vi "Peak Detector Comparison.vi"() -> ()   [LabVIEW 2020]
doc: "This VI compares the use of the Peak Detector.vi and the Peak Detector PtByPt.vi and how to use both VIs for the same problem. It also demonstrates how to use Data Queue PtByPt.vi to allow the function Peak Detector to work as a \"sliding window\" to find the location, amplitude, and second derivative of peaks or valleys in the set of generated input data."
uses:
  <vilib>/Analysis/1siggen.llb/Ramp Pattern by Samples.vi
  <vilib>/ptbypt/NI_PtbyPt.lvlib
  <vilib>/Analysis/NI_AALBase.lvlib
panel:
  in  "Motor Enable":bool
  out "First Peak":bool
  out "Motor":bool
  out "peak 2":bool
  in  "Noise Amplitude 2":dbl=1.0
  in  "Width 2":i32(slide)=10 min=3 scale=3.0..20.0
  in  "Sine Wave Amplitude 2":dbl=10.0
  out "peak":bool
  in  "Noise Amplitude":dbl=1.0
  in  "Stop":bool
  in  "Sine Wave Amplitude":dbl=10.0
  out "Signal Input and Peaks/Valleys from Peak Detector":cluster{"Locations":dbl[], "Amplitudes":dbl[]}[](graph)
  in  "Width":i32(slide)=10 min=3 scale=3.0..20.0
  in  "threshold":dbl(slide) scale=-15.0..15.0
  # "PtByPt Results"
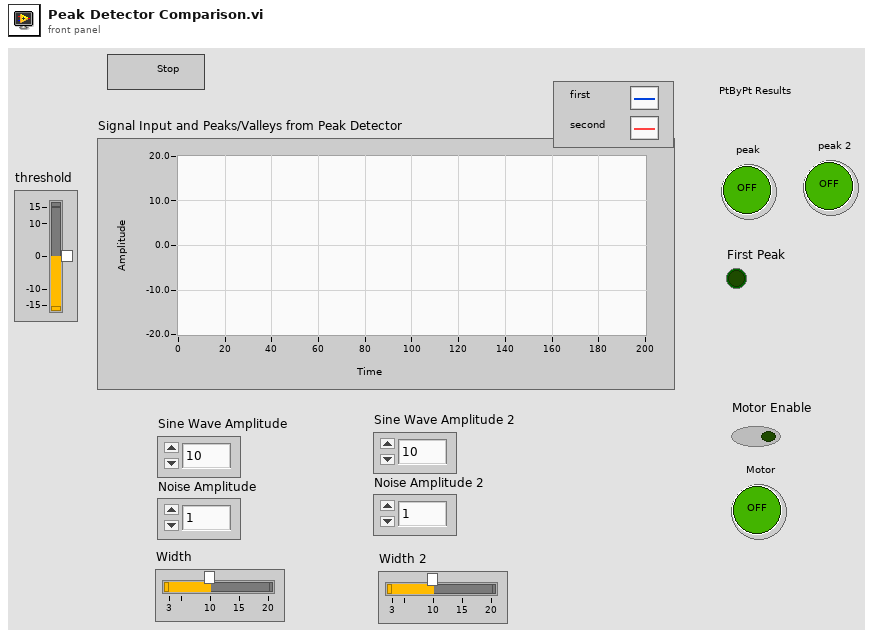
[diagram p1: front panel]
types:
  T1 = cluster{"Ramp Pattern":dbl[], "Current Queue":dbl[]}
  T2 = cluster{"Ramp Pattern":dbl[], "Current Queue":dbl[]}[]
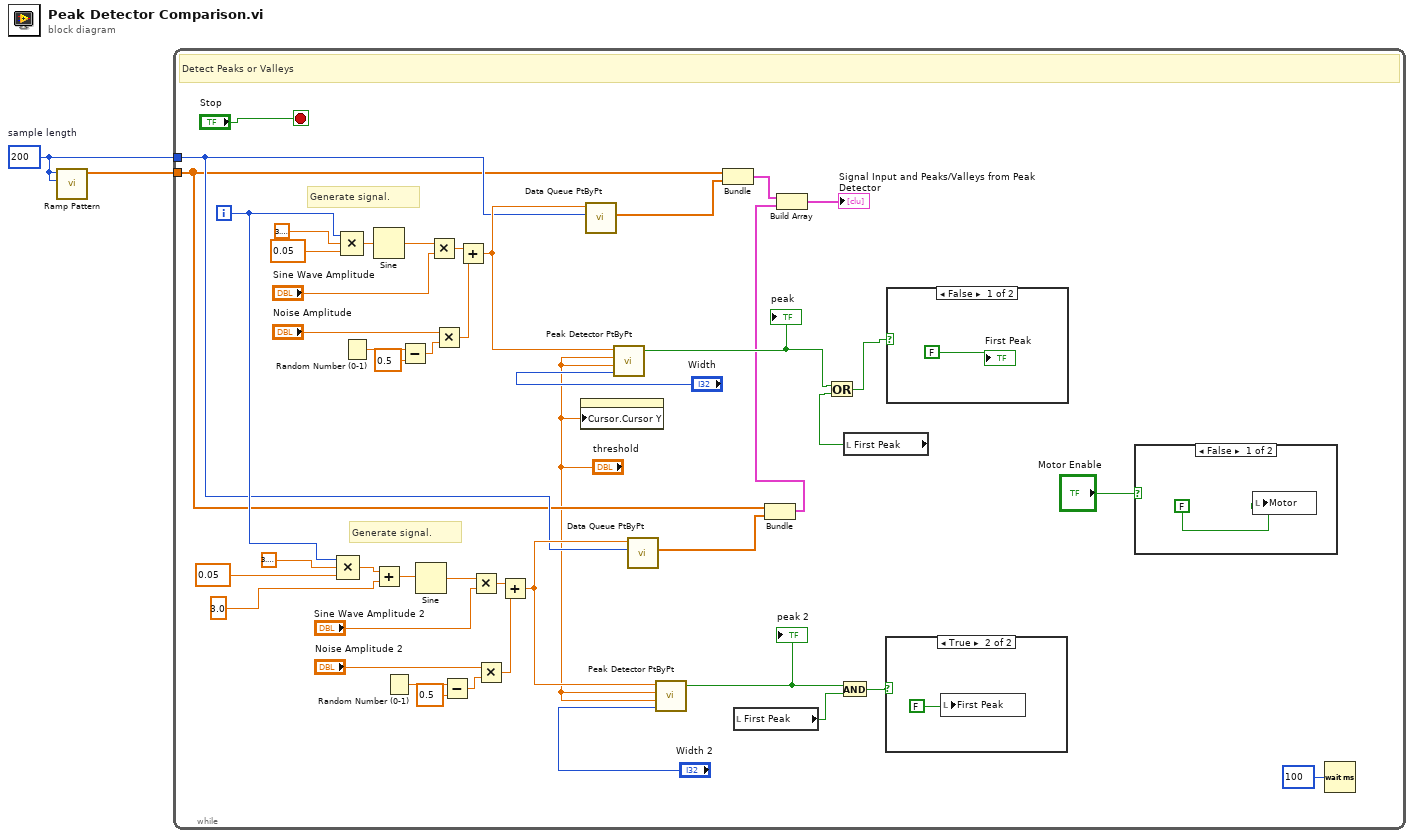
[diagram p0: block diagram]
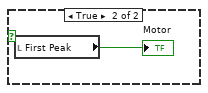
[diagram p2: hidden frame]
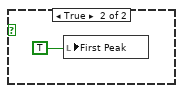
[diagram p4: hidden frame]
diagram:
  w1 = 200  # sample length
  n1 = call-poly <vilib>:"Ramp Pattern.vi"("end"=w1, "samples"=w1) -> ("Ramp Pattern"=w2:dbl[])  [unwired: 8 in, 1 out]
  n2 = while {
    tunnel: w1 -> [w16]
    tunnel: w2 -> [w15]
    i -> [w17]
    stop <- "Stop" stop-if-true
    # "Generate signal."
    # "Generate signal."
    # "Detect Peaks or Valleys"
    n3 = Compound Arithmetic op=MULTIPLY(w17, 3.141592653589793, 0.05 ("value")) -> (w11:dbl)
    n4 = Compound Arithmetic op=MULTIPLY(w17, 3.141592653589793, 0.05 ("value")) -> (w46:dbl)
    n5 = Random Number (0-1)() -> (number: 0 to 1=w39:dbl)
    n6 = Sine(x=w46) -> (sin(x)=w45:dbl)
    n7 = Add(x=w11, y=3.0) -> (x+y=w9:dbl)
    n8 = Random Number (0-1)() -> (number: 0 to 1=w24:dbl)
    n9 = Subtract(x=w39, y=0.5) -> (x-y=w38:dbl)
    n10 = Sine(x=w9) -> (sin(x)=w21:dbl)
    n11 = Multiply(x=w45, y="Sine Wave Amplitude") -> (x*y=w44:dbl)
    n12 = Multiply(x="Noise Amplitude", y=w38) -> (x*y=w37:dbl)
    n13 = Subtract(x=w24, y=0.5) -> (x-y=w25:dbl)
    n14 = Add(x=w44, y=w37) -> (x+y=w35:dbl)
    n15 = Multiply(x=w21, y="Sine Wave Amplitude 2") -> (x*y=w22:dbl)
    n16 = Multiply(x="Noise Amplitude 2", y=w25) -> (x*y=w26:dbl)
    n17 = Add(x=w22, y=w26) -> (x+y=w28:dbl)
    n18 = property on="Signal Input and Peaks/Valleys from Peak Detector" class="XYGraph (strict)"("Cursor.Cursor Y"="threshold") -> ()  [unwired: 2 in, 2 out]
    n19 = call <vilib>:"Data Queue PtByPt.vi"("sample length"=w16, "input data point"=w35) -> ("Current Queue"=w33:dbl[])  [unwired: 5 in, 4 out]
    n20 = call <vilib>:"Peak Detector PtByPt.vi"("x"=w35, "threshold peak"="threshold", "threshold valley"="threshold", "width"="Width") -> ("peak"=w13:bool)  [unwired: 1 in, 2 out]
    "peak" <- w13
    n21 = call <vilib>:"Data Queue PtByPt.vi"("sample length"=w16, "input data point"=w28) -> ("Current Queue"=w30:dbl[])  [unwired: 5 in, 4 out]
    n22 = call <vilib>:"Peak Detector PtByPt.vi"("x"=w28, "threshold peak"="threshold", "threshold valley"="threshold", "width"="Width 2") -> ("peak"=w5:bool)  [unwired: 1 in, 2 out]
    "peak 2" <- w5
    n23 = Bundle("Ramp Pattern"=w15, "Current Queue"=w33) -> (w47:T1)  [unwired: 1 out]
    n24 = local read "First Peak"() -> (w6:bool)
    n25 = Bundle("Ramp Pattern"=w15, "Current Queue"=w30) -> (w8:T1)  [unwired: 1 out]
    n26 = Build Array(w47, w8) -> (→"Signal Input and Peaks/Valleys from Peak Detector":T2)
    n27 = And(x=w5, y=w6) -> (x .and. y?=w4:bool)
    n28 = local read "First Peak"() -> (w14:bool)
    n29 = Or(x=w13, y=w14) -> (x .or. y?=w12:bool)
    n30 = case shown="True" w4 {
      frame False {
      }
      frame True {
        n31 = local write "First Peak"(FALSE) -> ()
      }
    }
    n32 = case shown="False" w12 {
      frame False {
        "First Peak" <- FALSE
      }
      frame True {
        n33 = local write "First Peak"(TRUE) -> ()
      }
    }
    n34 = case shown="False" "Motor Enable" {
      frame False {
        n35 = local write "Motor"(FALSE) -> ()
      }
      frame True {
        n36 = local read "First Peak"() -> (→"Motor":bool)
      }
    }
    n37 = Wait (ms)(milliseconds to wait=u32 100) -> ()  [unwired: 1 out]
  }
